vi "Notificador.vi"() -> ()   [LabVIEW 2019]
panel:
  out "notification":string
  in  "stop":bool
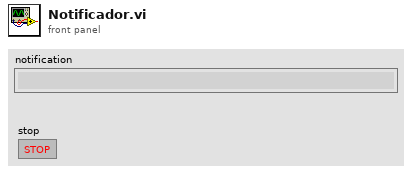
[diagram p1: front panel]
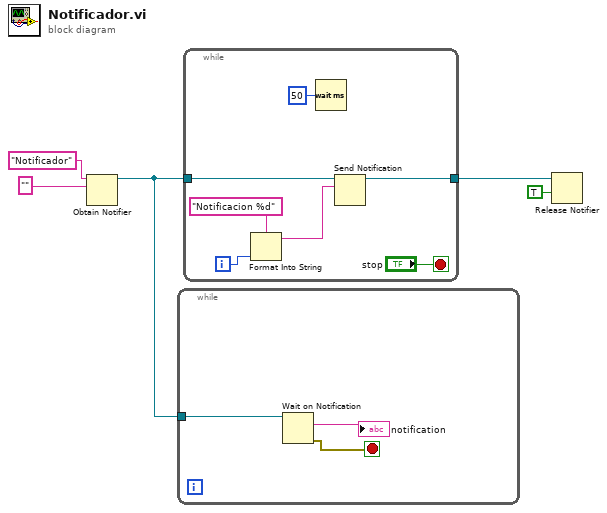
[diagram p0: block diagram]
diagram:
  n1 = Obtain Notifier(name (unnamed)="Notificador", notification data type="") -> (notifier out=w3:refnum<notifier>)  [unwired: 2 in, 2 out]
  n2 = while {
    tunnel: w3 -> [w6]
    stop <- w8 stop-if-true
    n3 = Wait on Notification(notifier=w6) -> (notification=→"notification":string, error out=w8:errorcluster)  [unwired: 3 in, 2 out]
  }
  n4 = while {
    tunnel: w3 -> [w12]
    tunnel: [w11] -> w5
    i -> [w15]
    stop <- "stop" stop-if-true
    n5 = Format Into String(format string="Notificacion %d", w15) -> (resulting string=w13:string)  [unwired: 2 in, 1 out]
    n6 = Wait (ms)(milliseconds to wait=u32 50) -> ()  [unwired: 1 out]
    n7 = Send Notification(notification=w13, notifier=w12) -> (notifier out=w11:refnum<notifier>)  [unwired: 1 in, 1 out]
  }
  n8 = Release Notifier(notifier=w5, force destroy? (F)=TRUE) -> ()  [unwired: 1 in, 3 out]
